vi "Primary Loop.vi"(6 "Pri Hot Temp (K)":dbl, 7 "Time Interval (s)":dbl, 8 "Pri Cold Temp (K)":dbl, 9 "Pri Mass Flow (kg/s) in":dbl, 10 "Reactor Power (W)":dbl, 11 "MHX Heat Transfer (W)":dbl) -> (0 "Pri Hot Temperature (K)":dbl, 1 "Pri Cold Temperature (K)":dbl, 2 "Pri Mass Flow (kg/s) out":dbl, 3 "Temperature (C) 2":dbl, 4 "Primary Average Temperature (C)":dbl, 5 "Temperature (C)":dbl)   [LabVIEW 2019]
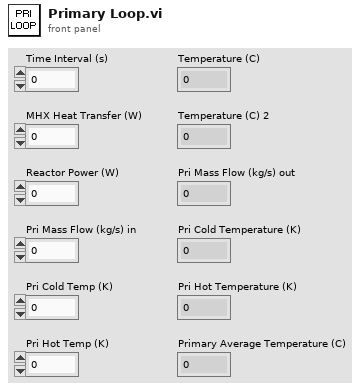
[diagram p1: front panel]
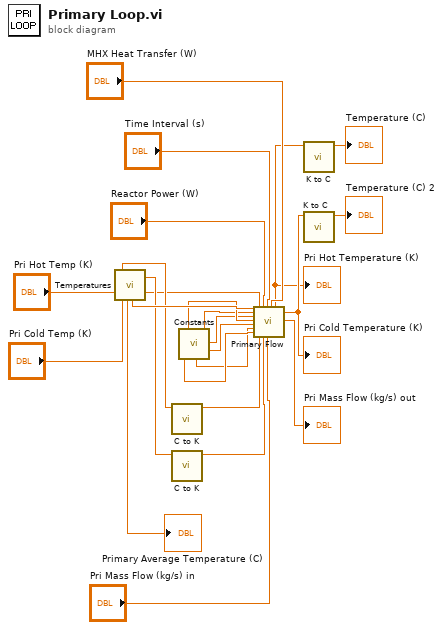
[diagram p0: block diagram]
diagram:
  n1 = call "Temperatures.vi"("Pri Hot Temp"="Pri Hot Temp (K)", "Pri Cold Temp"="Pri Cold Temp (K)") -> ("Primary Hot Temperature (C)"=w16:dbl, "Primary Average Temperature (C)"=→"Primary Average Temperature (C)":dbl, "Primary Delta T (K)"=w18:dbl, "Primary Cold Temperature (C)"=w15:dbl, "Primary Average Temperature (K)"=w14:dbl)  [unwired: 7 in, 6 out]
  n2 = call "C to K.vi"("Temperature (C)"=w16) -> ("Temperature (K)"=w7:dbl)  [unwired: 10 in]
  n3 = call "C to K.vi"("Temperature (C)"=w15) -> ("Temperature (K)"=w8:dbl)  [unwired: 10 in]
  n4 = call "Constants.vi"() -> ("MHX Tube Diameter (m)"=w4:dbl, "Pipe Diameter (m)"=w5:dbl, "MHX Length (m)"=w3:dbl, "Specific Heat Capacity of FLiBe (W/m-K)"=w1:dbl, "MHX Number of Tubes"=w2:dbl, "Pipe X-SectionArea (m^2)"=w6:dbl)  [unwired: 5 in, 17 out]
  n5 = call "Primary Flow.vi"("Primary Delta T"=w18, "Specific Heat Capacity of FLiBe"=w1, "MHX Number of Tubes"=w2, "Pipe Diameter"=w5, "Pipe X-SectionArea"=w6, "MHX Length"=w3, "MHX Tube Diameter"=w4, "Primary Average Temperature"=w14, "Pri Hot Temp"=w7, "Reactor Power"="Reactor Power (W)", "Pri Cold Temp"=w8, "Time Interval (s)"="Time Interval (s)", "Pri Mass Flow"="Pri Mass Flow (kg/s) in", "MHX Heat Transfer"="MHX Heat Transfer (W)") -> ("Pri Hot Temperature (K)"=w10:dbl, "Pri Cold Temperature (K)"=w12:dbl, "Pri Mass Flow (kg/s)"=→"Pri Mass Flow (kg/s) out":dbl)  [unwired: 5 in, 6 out]
  "Pri Cold Temperature (K)" <- w12
  "Pri Hot Temperature (K)" <- w10
  n6 = call "K to C.vi"("Temperature (K)"=w10) -> ("Temperature (C)"=→"Temperature (C)":dbl)  [unwired: 10 in]
  n7 = call "K to C.vi"("Temperature (K)"=w12) -> ("Temperature (C)"=→"Temperature (C) 2":dbl)  [unwired: 10 in]
